vi "create.vi"(8 "error in (no error)":errorcluster, 10 "Port":i32, 11 "ModbusFactory in":refnum<class "ModbusFactory.lvclass">) -> (0 "error out":errorcluster, 2 "Modbus":refnum<class "IModbus.lvclass">, 3 "ModbusFactory out":refnum<class "ModbusFactory.lvclass">)   [LabVIEW 2016, in "ModbusFactory.lvclass"]
uses:
  ModbusFactory.lvclass
  Common_RT_Modbus/IModbus/IModbus.lvclass
  ModbusFactory.lvclass/ModbusFactory.ctl
  Common_RT_Modbus/Modbus/Modbus.lvclass
  D:/Code/Common_RT_Modbus/IModbus/IModbus.lvclass
  ModbusPort1ReadFIFO/ModbusPort1ReadFIFO.lvclass
  D:/Code/Common_RT_FPGA/IReadU16FIFO/IReadU16FIFO.lvclass
  ModbusPort1WriteFIFO/ModbusPort1WriteFIFO.lvclass
  D:/Code/Common_RT_FPGA/IWriteU16FIFO/IWriteU16FIFO.lvclass
  SoftwareControlledTrigger/SoftwareControlledTrigger.lvclass
  D:/Code/Common_RT_FPGA/IBooleanControl/IBooleanControl.lvclass
  ModbusIRQs/ModbusIRQs.lvclass
  D:/Code/Common_RT_FPGA/IIRQ/IIRQ.lvclass
  ModbusPort1TimestampFIFO/ModbusPort1TimestampFIFO.lvclass
  D:/Code/Common_RT_FPGA/IReadU64FIFO/IReadU64FIFO.lvclass
  ModbusPort1TimestampFIFO/ModbusPort1TimestampFIFO.lvclass/ModbusPort1TimestampFIFO.ctl
  SoftwareControlledTrigger/SoftwareControlledTrigger.lvclass/SoftwareControlledTrigger.ctl
  ModbusPort1WriteFIFO/ModbusPort1WriteFIFO.lvclass/ModbusPort1WriteFIFO.ctl
  ModbusPort1ReadFIFO/ModbusPort1ReadFIFO.lvclass/ModbusPort1ReadFIFO.ctl
  Common_RT_Modbus/Modbus/Modbus.lvclass/Modbus.ctl
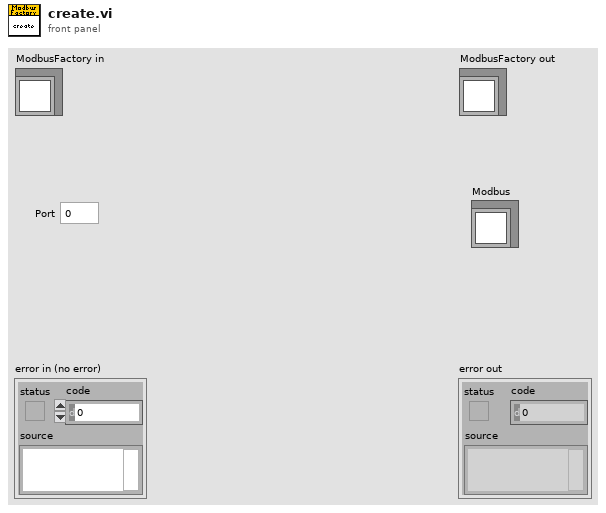
[diagram p1: front panel]
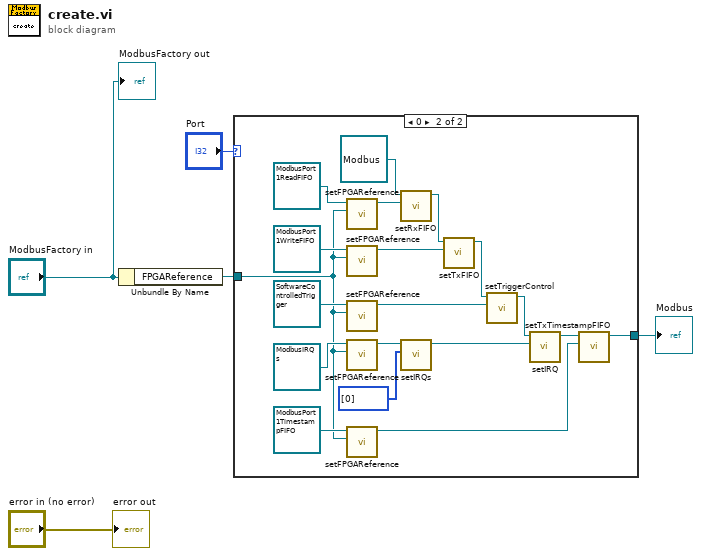
[diagram p0: block diagram]
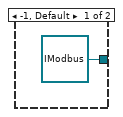
[diagram p2: hidden frame]
diagram:
  n1 = Unbundle By Name("ModbusFactory in") -> ("FPGAReference"=w4:refnum<k20>)
  n2 = case shown="0" "Port" {
    tunnel: w4 -> [_ w10]
    tunnel: [refnum<class "IModbus.lvclass"> refnum ("RTModbus.lvlib:IModbus.lvclass") w7] -> w3
    frame -1, Default {
    }
    frame 0 {
      n3 = call "setFPGAReference.vi"("FPGAReference"=w10, "ModbusPort1ReadFIFO in"=refnum<class "ModbusPort1ReadFIFO.lvclass"> refnum ("ModbusPort1ReadFIFO.lvclass")) -> ("ModbusPort1ReadFIFO out"=w23:refnum<class "ModbusPort1ReadFIFO.lvclass">)  [unwired: 9 in]
      n4 = call "setFPGAReference.vi"("FPGAReference"=w10, "ModbusPort1WriteFIFO in"=refnum<class "ModbusPort1WriteFIFO.lvclass"> refnum ("ModbusPort1WriteFIFO.lvclass")) -> ("ModbusPort1WriteFIFO out"=w21:refnum<class "ModbusPort1WriteFIFO.lvclass">)  [unwired: 9 in]
      n5 = call "setFPGAReference.vi"("FPGAReference"=w10, "SoftwareControlledTrigger in"=refnum<class "SoftwareControlledTrigger.lvclass"> refnum ("SoftwareControlledTrigger.lvclass")) -> ("SoftwareControlledTrigger out"=w18:refnum<class "SoftwareControlledTrigger.lvclass">)  [unwired: 9 in]
      n6 = call-dynamic "setFPGAReference.vi"("FPGAReference"=w10, "ModbusIRQs in"=refnum<class "ModbusIRQs.lvclass"> refnum ("ModbusIRQs.lvclass")) -> ("ModbusIRQs out"=w14:refnum<class "ModbusIRQs.lvclass">)  [unwired: 9 in]
      n7 = call "setFPGAReference.vi"("FPGAReference"=w10, "MyHealthAndStatusReadFIFO in"=refnum<class "ModbusPort1TimestampFIFO.lvclass"> refnum ("ModbusPort1TimestampFIFO.lvclass")) -> ("MyHealthAndStatusReadFIFO out"=w9:refnum<class "ModbusPort1TimestampFIFO.lvclass">)  [unwired: 9 in]
      n8 = call "setRxFIFO.vi"("ReadU16FIFO"=w23, "Modbus in"=refnum<class "Modbus.lvclass"> refnum ("RTModbus.lvlib:Modbus.lvclass")) -> ("Modbus out"=w20:refnum<class "Modbus.lvclass">)  [unwired: 9 in]
      n9 = call-dynamic "setIRQs.vi"("IRQs"=i32[] [0], "ModbusIRQs in"=w14) -> ("ModbusIRQs out"=w13:refnum<class "ModbusIRQs.lvclass">)  [unwired: 9 in]
      n10 = call "setTxFIFO.vi"("WriteU16FIFO"=w21, "Modbus in"=w20) -> ("Modbus out"=w17:refnum<class "Modbus.lvclass">)  [unwired: 9 in]
      n11 = call "setTriggerControl.vi"("BooleanControl"=w18, "Modbus in"=w17) -> ("Modbus out"=w15:refnum<class "Modbus.lvclass">)  [unwired: 9 in]
      n12 = call "setIRQ.vi"("IRQ"=w13, "Modbus in"=w15) -> ("Modbus out"=w8:refnum<class "Modbus.lvclass">)  [unwired: 9 in]
      n13 = call "setTxTimestampFIFO.vi"("TxTimestampFIFO"=w9, "Modbus in"=w8) -> ("Modbus out"=w7:refnum<class "Modbus.lvclass">)  [unwired: 9 in]
    }
  }
  "Modbus" <- w3
  "error out" <- "error in (no error)"
  "ModbusFactory out" <- "ModbusFactory in"
